vi "Initialize.vi"(8 "error in (no error)":errorcluster, 11 "Socket in":refnum<class "Socket.lvclass">) -> (0 "error out":errorcluster, 3 "Socket out":refnum<class "Socket.lvclass">)   [LabVIEW 2018, in "Socket.lvclass"]
uses:
  Socket.lvclass
  Socket.lvclass/Socket.ctl
  State Machine/State Machine.lvclass
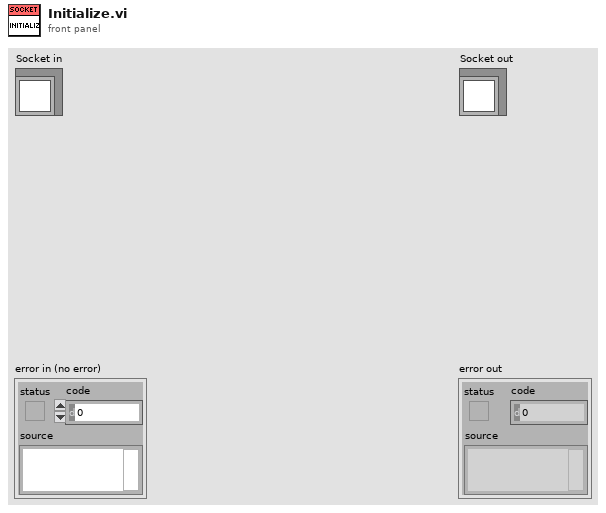
[diagram p1: front panel]
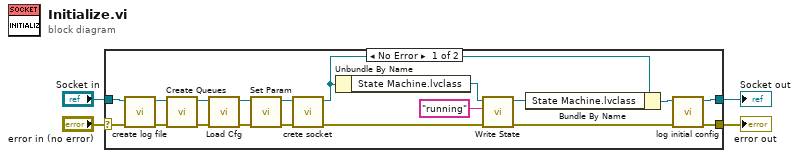
[diagram p0: block diagram]
diagram:
  n1 = case shown="No Error" "error in (no error)" {
    selector: "error in (no error)" -> [w9 w25]
    tunnel: [w6 w25] -> w3
    tunnel: [w7 w24] -> w1
    tunnel: "Socket in" -> [w12 w24]
    frame No Error {
      n2 = call "create log file.vi"("error in (no error)"=w9, "Socket in"=w12) -> ("error out"=w10:errorcluster, "Socket out"=w11:refnum<class "Socket.lvclass">)  [unwired: 8 in]
      n3 = call-dynamic "Create Queues.vi"("error in (no error)"=w10, "Socket in"=w11) -> ("error out"=w13:errorcluster, "Socket out"=w14:refnum<class "Socket.lvclass">)  [unwired: 8 in]
      n4 = call-dynamic "Load Cfg.vi"("error in (no error)"=w13, "Socket in"=w14) -> ("error out"=w17:errorcluster, "Socket out"=w20:refnum<class "Socket.lvclass">)  [unwired: 8 in]
      n5 = call-dynamic "Set Param.vi"("error in (no error)"=w17, "Socket in"=w20) -> ("error out"=w16:errorcluster, "Socket out"=w19:refnum<class "Socket.lvclass">)  [unwired: 8 in]
      n6 = call "crete socket.vi"("error in (no error)"=w16, "Socket in"=w19) -> ("error out"=w15:errorcluster, "Socket out"=w18:refnum<class "Socket.lvclass">)  [unwired: 8 in]
      n7 = Unbundle By Name(w18) -> ("State Machine.lvclass"=w22:refnum<class "State Machine.lvclass">)
      n8 = call-dynamic "Write State.vi"("error in (no error)"=w15, "State"="running", "State Machine in"=w22) -> ("error out"=w5:errorcluster, "State Machine out"=w21:refnum<class "State Machine.lvclass">)  [unwired: 7 in]
      n9 = Bundle By Name(cluster=w18, "State Machine.lvclass"=w21) -> (w8:refnum<class "Socket.lvclass">)
      n10 = call "log initial config.vi"("error in (no error)"=w5, "Socket in"=w8) -> ("error out"=w6:errorcluster, "Socket out"=w7:refnum<class "Socket.lvclass">)  [unwired: 8 in]
    }
    frame Error {
    }
  }
  "error out" <- w3
  "Socket out" <- w1
